vi "Method.vi"(4 "Value":refnum<class "Abs_I8 Integer.lvclass">) -> (1 "Result":refnum<class "Abs_I8 Integer.lvclass">)   [LabVIEW 2021, in "Invert_I8.lvclass"]
uses:
  Invert_I8.lvclass
  Abs_Types/I8 Integer/Abs_I8 Integer.lvclass
  C:/TSA/LV_Abstract/Source/Functions/Support/Function/One Terminal/I8/AbsFunc_One Term_I8.lvclass
  C:/Program Files (x86)/National Instruments/LabVIEW 2021/vi.lib/TSA/Abstract Data Classes/Abs_Types/I8 Integer/Abs_I8 Integer.lvclass
  Support/Function/One Terminal/I8/AbsFunc_One Term_I8.lvclass/AbsFunc_One Term_I8.ctl
  Support/Function/One Terminal/I8/Properties/Write Numeric A.vi
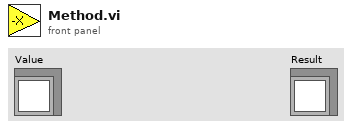
[diagram p1: front panel]
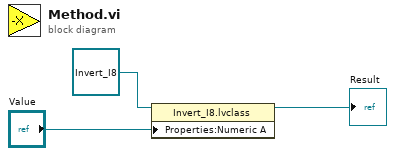
[diagram p0: block diagram]
diagram:
  n1 = property class="Invert_I8.lvclass"(reference=refnum<class "Invert_I8.lvclass"> refnum ("Invert_DBL.lvclass"), "Properties:Numeric A"="Value") -> (reference out=→"Result":refnum<class "Invert_I8.lvclass">)  [unwired: 1 in, 1 out]
